vi "Log Error.vi"(8 "error in (no error)":errorcluster, 10 "Error Message Data":T1, 11 "Error Handler In":refnum<class "Error Handler.lvclass">) -> (0 "error out":errorcluster, 3 "Error Handler Out":refnum<class "Error Handler.lvclass">)   [LabVIEW 2020, in "Error Handler.lvclass"]
uses:
  Error Handler.lvclass
  Public/TypeDefs/Error Message Data.ctl
  Error Handler.lvclass/Error Handler.ctl
  Support/Error Log Classes/Error Log/Error Log.lvclass
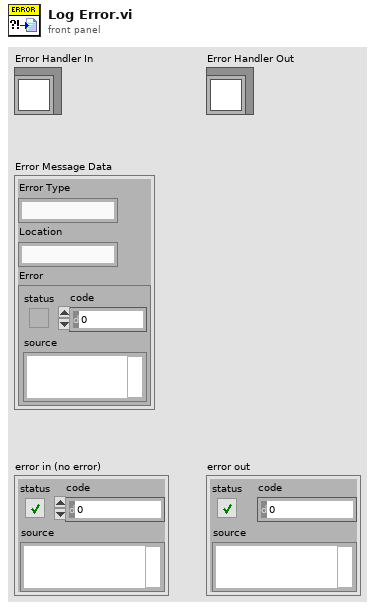
[diagram p1: front panel]
types:
  T1 = typedef "Error Handler.lvclass/Error Message Data.ctl" = cluster{"Error Type":string, "Location":string, "Error":errorcluster}
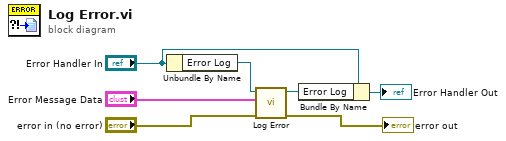
[diagram p0: block diagram]
diagram:
  n1 = Unbundle By Name("Error Handler In") -> ("Error Log"=w1:refnum<class "Error Log.lvclass">)
  n2 = call-dynamic "Log Error.vi"("error in (no error)"="error in (no error)", "Error Message Data"="Error Message Data", "Error Log In"=w1) -> ("error out"=→"error out":errorcluster, "Error Log Out"=w2:refnum<class "Error Log.lvclass">)  [unwired: 7 in]
  n3 = Bundle By Name(cluster="Error Handler In", "Error Log"=w2) -> (→"Error Handler Out":refnum<class "Error Handler.lvclass">)
